vi "Date Time String to Seconds_RageATE.vi"(6 "DST":bool, 11 "Time/date(str)in":string="11:34:38 AM 4/4/2023 ") -> (1 "Timestamp from Number of Seconds":timestamp, 2 "Number of Seconds":dbl, 3 "Timestamp from Date/Time String":timestamp)   [LabVIEW 2018]
doc: "This example is used to convert a date and time string back into a timestamp."
uses:
  <vilib>/Utility/miscctls.llb/LVDateTimeRec.ctl
panel:
  # "Overview: This example is used to convert a date and time string back into a timestamp.\nRequirements: LabVIEW 2012 (or compatible)\nInstructions:\nRun the VI and the conversation results will display on Front Panel."
  # "Derived/Computed Values"
  # "Note: the only thing that's off is the Fractional Seconds, but that's because you don't have that information\nin the date/time string"
  # "4/3/2023 7:16 PM"
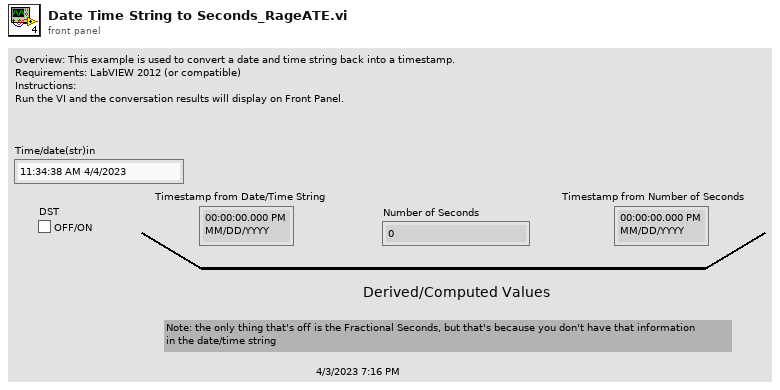
[diagram p1: front panel]
types:
  T1 = typedef "LVDateTimeRec.ctl" = cluster{"fractional second":dbl, "second":i32, "minute":i32, "hour":i32, "day of month":i32, "month":i32, "year":i32, "day of week":i32, "day of year":i32, "DST":i32}
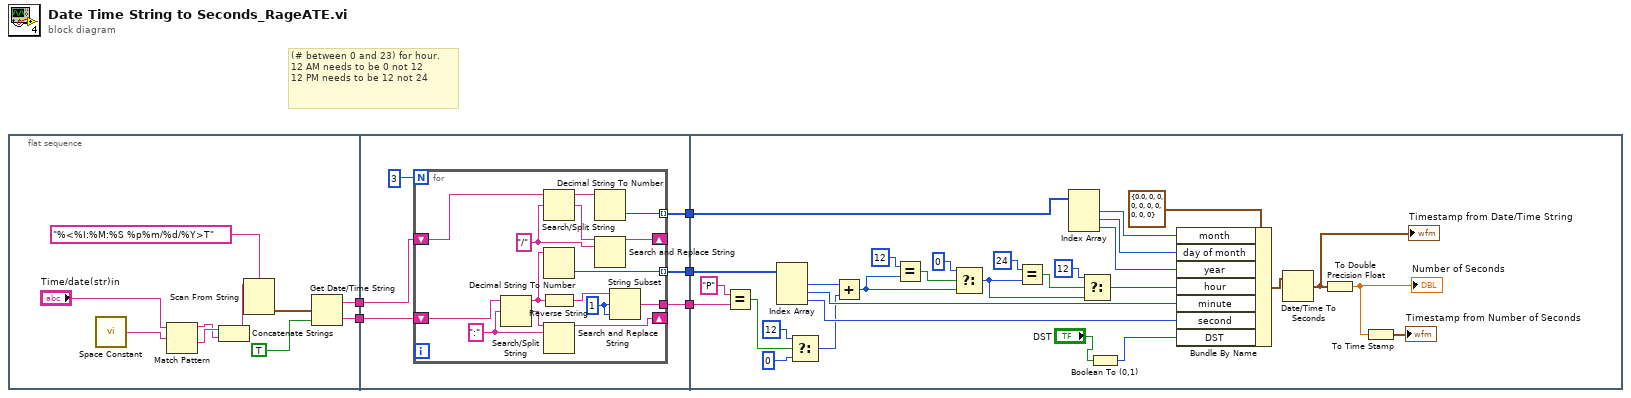
[diagram p0: block diagram]
diagram:
  # "(# between 0 and 23) for hour.\n12 AM needs to be 0 not 12\n12 PM needs to be 12 not 24"
  n1 = flat-sequence {
    tunnel: [w11] -> w2
    tunnel: [w12] -> w1
    tunnel: [w18] -> w5
    tunnel: [w17] -> w4
    tunnel: [w16] -> w3
    tunnel: w2 -> [w20]
    tunnel: w1 -> [w19]
    tunnel: w5 -> [w40]
    tunnel: w4 -> [w41]
    tunnel: w3 -> [w45]
    frame #0 {
      n2 = call <vilib>:"Space Constant.vi"() -> ("String"=w10:string)
      n3 = Match Pattern(string="Time/date(str)in", regular expression=w10) -> (before substring=w8:string, after substring=w9:string)  [unwired: 1 in, 2 out]
      n4 = Concatenate Strings(w9, w8) -> (w6:string)
      n5 = Scan From String(format string="%<%I:%M:%S %p%m/%d/%Y>T", input string=w6) -> (output 1=w15:timestamp)  [unwired: 3 in, 3 out]
      n6 = Get Date/Time String(seconds (now)=w15, want seconds? (F)=TRUE) -> (date string=w11:string, time string=w12:string)  [unwired: 1 in]
    }
    frame #1 {
      n7 = for {
        N: 3 -> [_]
        shift-right: [w34] -> _
        shift-left: w20 -> [w35]
        tunnel: [w32] -> w16 mode=indexing
        shift-right: [w31] -> _
        shift-left: w19 -> [w27]
        tunnel: [w28] -> w17 mode=indexing
        tunnel: [w22] -> w18
        w23 = 1 ("offset (0)")
        w29 = ":" ("search string/char (-)")
        w30 = "/" ("search string/char (-)")
        n8 = Search/Split String(string=w27, search string/char (-)=w29) -> (substring before match=w25:string, match + rest of string=w26:string)  [unwired: 1 in, 1 out]
        n9 = Search/Split String(string=w35, search string/char (-)=w30) -> (substring before match=w33:string, match + rest of string=w36:string)  [unwired: 1 in, 1 out]
        n10 = Decimal String To Number(string=w25) -> (number=w28:i32)  [unwired: 2 in, 1 out]
        n11 = Reverse String(1:w25) -> (0:w24:string)
        n12 = Search and Replace String(input string=w26, search string=w29) -> (result string=w31:string)  [unwired: 6 in, 3 out]
        n13 = Decimal String To Number(string=w33) -> (number=w32:i32)  [unwired: 2 in, 1 out]
        n14 = Search and Replace String(input string=w36, search string=w30) -> (result string=w34:string)  [unwired: 6 in, 3 out]
        n15 = String Subset(string=w24, offset (0)=w23, length (rest)=w23) -> (substring=w22:string)
      }
    }
    frame #2 {
      n16 = Equal?(x="P", y=w40) -> (x = y?=w50:bool)
      n17 = Index Array(array=w41) -> (element #1=w52:i32, element #2=w56:i32, element #3=w57:i32)  [unwired: 3 in]
      n18 = Select(t=12 ("index"), s=w50, f=0 ("index")) -> (s? t:f=w51:i32)
      n19 = Add(x=w52, y=w51) -> (x+y=w61:i32)
      n20 = Equal?(x=12 ("y"), y=w61) -> (x = y?=w60:bool)
      n21 = Select(t=0, s=w60, f=w61) -> (s? t:f=w62:i32)
      n22 = Equal?(x=24 ("y"), y=w62) -> (x = y?=w59:bool)
      n23 = Index Array(array=w45) -> (element #1=w53:i32, element #2=w54:i32, element #3=w55:i32)  [unwired: 3 in]
      n24 = Select(t=12 ("index"), s=w59, f=w62) -> (s? t:f=w63:i32)
      n25 = Boolean To (0,1)(Boolean="DST") -> (0, 1=w38:i16)
      n26 = Bundle By Name(cluster=T1 {"fractional second"=0.0, "second"=0, "minute"=0, "hour"=0, "day of month"=0, "month"=0, "year"=0, "day of week"=0, "day of year"=0, "DST"=0} ("date time rec"), "month"=w53, "day of month"=w54, "year"=w55, "hour"=w63, "minute"=w56, "second"=w57, "DST"=w38) -> (w58:T1)
      n27 = Date/Time To Seconds(2:w58) -> (0:w64:timestamp)  [unwired: 1 in]
      "Timestamp from Date/Time String" <- w64
      n28 = To Double Precision Float(number=w64) -> (double precision float=w65:dbl)
      "Number of Seconds" <- w65
      n29 = To Time Stamp(1:w65) -> (0:→"Timestamp from Number of Seconds":timestamp)
    }
  }
